vi "Read.vi"(11 "GroupsValue in":refnum<class "GroupArrayValue.lvclass">) -> (2 "Groups":refnum<class "Group DBL.lvclass">[](array[class]))   [LabVIEW 2020, in "Vecto.lvlib" / "GroupArrayValue.lvclass"]
uses:
  GroupArrayValue.lvclass
  Group DBL/Group DBL.lvclass
  GroupArrayValue.lvclass/GroupArrayValue.ctl
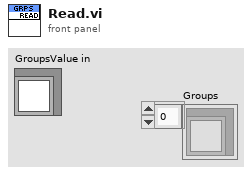
[diagram p1: front panel]
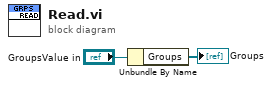
[diagram p0: block diagram]
diagram:
  n1 = Unbundle By Name("GroupsValue in") -> ("Groups"=→"Groups":refnum<class "Group DBL.lvclass">[])
